vi "Mode Selector.vi"(9 "Middle Mode Off":bool, 11 "Middle Mode On":bool) -> ()   [LabVIEW 2012]
panel:
  out "Middle Mode?":bool=TRUE
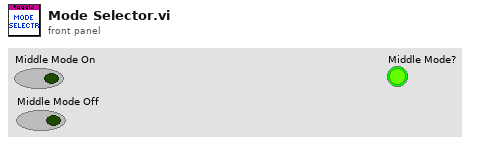
[diagram p1: front panel]
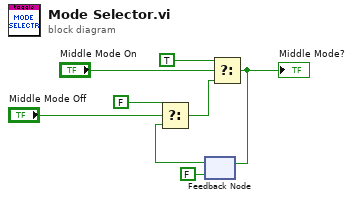
[diagram p0: block diagram]
diagram:
  n1 = feedback #1(FALSE) -> (w5:bool)
  n2 = Select(t=FALSE, s="Middle Mode Off", f=w5) -> (s? t:f=w6:bool)
  n3 = Select(t=TRUE, s="Middle Mode On", f=w6) -> (s? t:f=w2:bool)
  "Middle Mode?" <- w2
  n4 = feedback-in #1(w2) -> ()
